vi "Esercitazione 3 - Somma4 SubVI.vi"(1 "Numeric Control 4":dbl, 2 "Numeric Control 3":dbl, 3 "Numeric Control 2":dbl, 4 "Numeric Control":i32) -> (0 "Numeric Indicator":dbl)   [LabVIEW 2018]
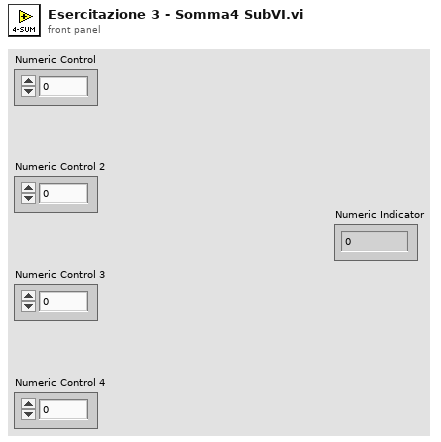
[diagram p1: front panel]
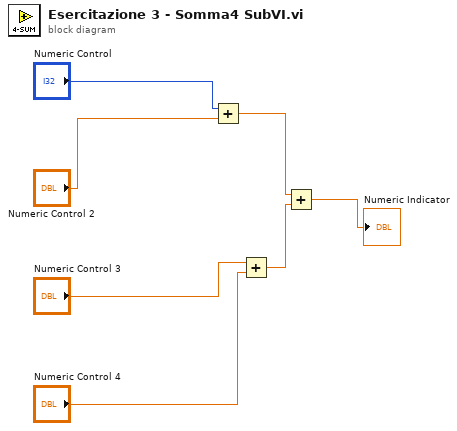
[diagram p0: block diagram]
diagram:
  n1 = Add(x="Numeric Control", y="Numeric Control 2") -> (x+y=w3:dbl)
  n2 = Add(x="Numeric Control 3", y="Numeric Control 4") -> (x+y=w2:dbl)
  n3 = Add(x=w3, y=w2) -> (x+y=→"Numeric Indicator":dbl)
